vi "监控电脑运行信息vi.vi"() -> ()   [LabVIEW 2025]
uses:
  <vilib>/nisyscfg/File System.ctl
  <vilib>/nisyscfg/Access Point.ctl
  <vilib>/nisyscfg/Wireless Network.ctl
  <vilib>/nisyscfg/Resource Expert Info.ctl
  <resource>/objmgr/nicontrollersysapi.rc
  <resource>/objmgr/nisysapi.rc
  <vilib>/nisyscfg/nisyscfg.lvlib
panel:
  out "输出簇 2":T4 {"网络适配器:无线:发现接入点"."wireless network"."security type" items=["无"=0, "开环"=2, "WEP"=4, "WPA Personal"=8, "WPA Enterprise"=16, "WPA2 Personal"=32, "WPA2 Enterprise"=64]; "网络适配器:无线:发现接入点"."wireless network"."connection type" items=["无", "基础结构", "ad hoc"]; "网络适配器:无线:发现接入点"."link speed" items=["无"=0, "自适应"=1, "10mbps/半双工"=2, "10mbps/全双工"=4, "100mbps/半双工"=8, "100mbps/全双工"=16, "Gigabit/半双工"=32, "Gigabit/全双工"=64, "WLAN 802.11a"=131072, "WLAN 802.11b"=262144, "WLAN 802.11g"=524288, "WLAN 802.11n"=1048576, "WLAN 802.11n (5GHz)"=2097152]}
  in  "簇 2":T4={"系统硬件输出"=refnum, "错误输出"={"status"=FALSE, "code"=0, "source"=""}, "Startup Settings:Enable Secure Shell Server"=FALSE, "Startup Settings:Disable RT Startup App"=FALSE, "Startup Settings:Enable UI Desktop Environment"=FALSE, "Startup Settings:Enable LabVIEW Project Access"=FALSE, "属于设备"=FALSE, "属于机箱"=FALSE, "服务类型"=[], "设备与机箱:连接至总线类型"=0, "设备与机箱:提供总线类型"=0, "设备与机箱:供应商名称"="", "设备与机箱:产品名称"="", "设备与机箱:型号名称号"=0, "设备与机箱:序列号"="", "设备与机箱:属于NI产品"=FALSE, "设备与机箱:属于仿真"=FALSE, "设备与机箱:连接至链接名称"="", "设备与机箱:提供链接名称"="", "设备与机箱:插槽连接数"=0, "设备与机箱:提供插槽数"=0, "设备与机箱:插槽号"=0, "设备与机箱:插槽左偏移"=0, "设备与机箱:当前温度"=0.0, "设备与机箱:硬件版本"="", "设备与机箱:包含驱动"=-1, "设备与机箱:已存在"=-2, "设备与机箱:总线特定:供应商ID"=0, "设备与机箱:总线特定:产品ID"=0, "设备与机箱:总线特定:PXI/PCI总线数"=0, "设备与机箱:总线特定:PXI/PCI设备数"=0, "设备与机箱:总线特定:PXI/PCI函数数"=0, "设备与机箱:总线特定:PXI/PCI实际链接宽度"=0, "设备与机箱:总线特定:PXI/PCI最大链接宽度"=0, "设备与机箱:总线特定:USB接口"=0, "设备与机箱:总线特定:TCP/IP主机名称"="", "设备与机箱:总线特定:TCP/IP MAC地址"="", "设备与机箱:总线特定:TCP/IP地址"="", "设备与机箱:总线特定:TCP/IP设备类"="", "设备与机箱:总线特定:GPIB主地址"=0, "设备与机箱:总线特定:GPIB次地址"=0, "设备与机箱:总线特定:串行COM端口绑定"="", "设备与机箱:总线特定:cRIO模块编程模式"=0, "设备与机箱:外部校准:支持外部校准"=FALSE, "设备与机箱:外部校准:支持校准写入"=FALSE, "设备与机箱:外部校准:校准注释"="", "设备与机箱:外部校准:外部校准日期"=timestamp(0 s since 1904-01-01), "设备与机箱:外部校准:外部校准调整日期"=timestamp(0 s since 1904-01-01), "设备与机箱:外部校准:外部校准温度"=0.0, "设备与机箱:外部校准:外部校准截止日期"=timestamp(0 s since 1904-01-01), "设备与机箱:外部校准:推荐校准间隔"=0, "设备与机箱:外部校准:外部校准有限"=FALSE, "设备与机箱:外部校准:校准Checksum"="", "设备与机箱:内部校准:支持内部校准"=FALSE, "设备与机箱:内部校准:内部校准有限"=FALSE, "设备与机箱:内部校准:范围内内部校准值"=FALSE, "设备与机箱:内部校准:内部校准详细信息计数"=0, "设备与机箱:内部校准:内部校准名称"=[], "设备与机箱:内部校准:内部校准日期"=[], "设备与机箱:内部校准:内部校准温度"=[], "设备与机箱:固件:固件版本"="", "设备与机箱:固件:支持固件更新"=FALSE, "设备与机箱:固件:固件更新模式"=0, "设备与机箱:固件:固件文件匹配模式"="", "设备与机箱:固件:可用固件版本"=[], "设备与机箱:功能激活:功能激活状态"=0, "设备和机箱:功能激活:已激活功能的数量"=0, "设备和机箱:功能激活:已激活功能的名称"=[], "设备和机箱:功能激活:已激活功能的ID"=[], "启动设置:用户指定型安全模式"=FALSE, "启动设置:启用控制台输出"=FALSE, "启动设置:IP重置"=FALSE, "网络适配器:适配器类型"=1, "网络适配器:MAC地址"="", "网络适配器:属于主适配器"=FALSE, "网络适配器:适配器模式"=1, "网络适配器:TCP/IP:IP地址请求模式"=1, "网络适配器:TCP/IP:IP地址"="", "网络适配器:TCP/IP:子网掩码"="", "网络适配器:TCP/IP:网关"="", "网络适配器:TCP/IP:DNS服务器"="", "网络适配器:TCP/IP:当前链接速度"=1, "网络适配器:TCP/IP:包检测"=1, "网络适配器:TCP/IP:轮询间隔"=0, "网络适配器:无线:发现接入点"=[], "网络适配器:无线:SSID"="", "网络适配器:无线:连接类型"=0, "网络适配器:无线:安全类型"=0, "网络适配器:无线:链接质量"=0, "网络适配器:无线:通道编号"=0, "网络适配器:无线:BSSID"="", "网络适配器:无线:国家代码"=0, "网络适配器:无线:认证类型"=0, "系统资源:主磁盘空间"=0.0, "系统资源:剩余主磁盘空间"=0.0, "系统资源:CPU:CPU核心数量"=0, "系统资源:CPU:CPU逻辑处理器数量"=0, "系统资源:CPU:模型"="", "系统资源:CPU:步进修订"=0, "系统资源:CPU:总负载"=[], "系统资源:CPU:中断负载"=[], "系统资源:CPU:速度"=[], "系统资源:风扇:数量"=0, "系统资源:风扇:名称"=[], "系统资源:风扇:读数"=[], "系统资源:内存:物理内存总数"=0.0, "系统资源:内存:剩余物理内存"=0.0, "系统资源:内存:最大可用内存块"=0.0, "系统资源:内存:虚拟内存总数"=0.0, "系统资源:内存:剩余虚拟内存"=0.0, "系统资源:功率传感器:数量"=0, "系统资源:功率传感器:名称"=[], "系统资源:功率传感器:读数"=[], "系统资源:功率传感器:高临界值"=[], "系统资源:温度传感器:数量"=0, "系统资源:温度传感器:名称"=[], "系统资源:温度传感器:读数"=[], "系统资源:温度传感器:低临界值"=[], "系统资源:温度传感器:高临界值"=[], "系统资源:User LED:数量"=0, "系统资源:User LED:名称"=[], "系统资源:User LED:状态"=[], "系统资源:用户开关:数量"=0, "系统资源:用户开关:名称"=[], "系统资源:用户开关:状态"=[], "系统资源:电压传感器:数量"=0, "系统资源:电压传感器:名称"=[], "系统资源:电压传感器:读数"=[], "系统资源:电压传感器:额定值"=[], "系统资源:电压传感器:低临界值"=[], "系统资源:电压传感器:高临界值"=[], "时间:系统开始时间"=timestamp(0 s since 1904-01-01), "时间:当前时间"=timestamp(0 s since 1904-01-01), "时间:时区"="", "专项软件信息:专项软件名称"="", "专项软件信息:资源名称"="", "专项软件信息:用户别名"="", "专项软件信息:全部专项软件"=[], "System Resources:Memory Module:Location"=[], "System Resources:Memory Module:Model Name"=[], "System Resources:Memory Module:Capacity"=[], "System Resources:Fans:PXI Chassis Fan Control:Fan Mode"=1, "System Resources:Fans:PXI Chassis Fan Control:Fan User RPM"=0, "System Resources:Fans:PXI Chassis Fan Control:Fan User Duty Cycle"=0, "System Resources:Fans:PXI Chassis Fan Control:Fan User RPM Low Bound"=0, "System Resources:Fans:PXI Chassis Fan Control:Fan User RPM High Bound"=0, "System Resources:Fans:PXI Chassis Fan Control:Cooling Profile"=1, "System Resources:Fans:PXI Chassis Fan Control:Cooling Profile Source"=-1, "System Resources:Fans:PXI Chassis Fan Control:Enable User Override of Cooling Profile"=FALSE, "System Resources:Power Supplies:Count"=0, "System Resources:Power Supplies:Redundant"=0, "System Resources:Power Supplies:Bay Names"=[], "System Resources:Power Supplies:State"=[], "System Resources:Power Supplies:Max Power"=[], "System Resources:Power Supplies:Power Reading"=[], "System Resources:Power Supplies:Intake Temperature"=[], "System Resources:Power Supplies:Power Line Frequency"=[], "System Resources:Power Supplies:Inhibit Mode"=1, "Devices & Chassis:Bus Specific:PXI Chassis Number"=0, "Devices & Chassis:Bus Specific:PXI CLK10 Source"=-1, "Devices & Chassis:Bus Specific:External Clock Output Source"=-1, "Devices & Chassis:Bus Specific:Internal Oscillator"=-1, "Devices & Chassis:Bus Specific:High Density Trig Ports:Count"=0, "Devices & Chassis:Bus Specific:High Density Trig Ports:Names"=[], "Devices & Chassis:Bus Specific:High Density Trig Ports:States"=[], "Devices & Chassis:Bus Specific:High Density Trig Ports:Remote Aliases"=[], "Devices & Chassis:Bus Specific:Chassis LED Blink Pattern"=1, "Devices & Chassis:Calibration:PXI Chassis External Calibration Action"=0, "Devices & Chassis:Calibration:PXI Chassis Oscillator DAC Value"=0} {"Devices & Chassis:Calibration:PXI Chassis External Calibration Action" items=["Cancel", "OCXO Start", "Commit"]; "Devices & Chassis:Bus Specific:Chassis LED Blink Pattern" items=["Chassis Controlled"=1, "Blink"=2, "Blink | Blink | Blink"=4, "Blink | Blink | Steady"=8, "Blink | Steady | Blink"=16, "Blink | Steady | Steady"=32, "Steady | Blink | Blink"=64, "Steady | Blink | Steady"=128, "Steady | Steady | Blink"=256]; "Devices & Chassis:Bus Specific:High Density Trig Ports:States" items=["Disconnected", "Connected", "Connected (Off-Host)", "Loopback (Invalid)"]; "Devices & Chassis:Bus Specific:Internal Oscillator" items=["Unsupported"=-1, "VCXO"=0, "OCXO"=1]; "Devices & Chassis:Bus Specific:External Clock Output Source" items=["Unknown"=-1, "PXI_CLK10"=0, "Internal Oscillator"=1]; "Devices & Chassis:Bus Specific:PXI CLK10 Source" items=["Unknown"=-1, "Internal"=0, "10 MHz REF IN"=1, "Timing Module"=2, "TRIG / 10 MHz Port 0"=3]; "System Resources:Power Supplies:Inhibit Mode" items=["Default (Power Button/OS)"=1, "Manual (Remote Inhibit)"=2]; "System Resources:Power Supplies:State" items=["Off"=0, "On"=1, "Faulted"=2, "Fault: 12V Output Voltage Exceeded Upper Critical Limit"=16, "Fault: 12V Output Voltage Exceeded Lower Critical Limit"=17, "Fault: 5V Aux Output Voltage Exceeded Upper Critical Limit"=18, "Fault: 5V Aux Output Voltage Exceeded Lower Critical Limit"=19, "Fault: 12V Output Current Exceeded Critical Limit"=20, "Fault: 5V Aux Output Current Exceeded Critical Limit"=21, "Fault: AC Input Voltage Exceeded Upper Critical Limit"=22, "Fault: AC Input Voltage Exceeded Lower Critical Limit"=23, "Fault: Intake Temperature Exceeded Lower Critical Limit"=24, "Fault: Intake Temperature Exceeded Upper Critical Limit"=25, "Fault: Internal Temperature Exceeded Lower Critical Limit"=26, "Fault: Internal Temperature Exceeded Upper Critical Limit"=27, "Fault: Critical Fan Failure"=28, "Alert: 12V Output Voltage Exceeded Upper Alert Limit"=48, "Alert: 12V Output Voltage Exceeded Lower Alert Limit"=49, "Alert: 5V Aux Output Voltage Exceeded Upper Alert Limit"=50, "Alert: 5V Aux Output Voltage Exceeded Lower Alert Limit"=51, "Alert: 12V Output Current Exceeded Alert Limit"=52, "Alert: 5V Aux Output Current Exceeded Alert Limit"=53, "Alert: Current Sharing"=54, "Alert: AC Input Voltage Exceeded Upper Alert Limit"=55, "Alert: AC Input Voltage Exceeded Lower Alert Limit"=56, "Alert: Intake Temperature Exceeded Lower Alert Limit"=57, "Alert: Intake Temperature Exceeded Upper Alert Limit"=58, "Alert: Internal Temperature Exceeded Lower Alert Limit"=59, "Alert: Internal Temperature Exceeded Upper Alert Limit"=60, "Alert: Fan Failure"=61]; "System Resources:Power Supplies:Redundant" items=["Not Redundant", "Redundant"]; "System Resources:Fans:PXI Chassis Fan Control:Cooling Profile Source" items=["Unknown"=-1, "User Specified"=1, "Module Request"=2, "User Override of Module Request"=3]; "System Resources:Fans:PXI Chassis Fan Control:Cooling Profile" items=["38W"=1, "58W"=2, "82W"=4]; "System Resources:Fans:PXI Chassis Fan Control:Fan Mode" items=["Auto"=1, "Safe Manual"=2, "High"=4]; "系统资源:用户开关:状态" items=["Disabled", "已启用"]; "系统资源:User LED:状态" items=["Off"=0, "绿灯常亮"=1, "黄灯常亮"=2, "红灯常亮"=16, "绿灯闪烁"=4, "黄灯闪烁"=8, "红灯闪烁"=32]; "网络适配器:无线:认证类型" items=["None"=0, "EAP-TLS"=1, "EAP-TTLS"=2, "EAP-FAST"=4, "LEAP"=8, "PEAP"=16]; "网络适配器:无线:安全类型" items=["None"=0, "不支持"=1, "打开"=2, "WEP"=4, "WPA PSK"=8, "WPA EAP"=16, "WPA2 PSK"=32, "WPA2 EAP"=64]; "网络适配器:无线:连接类型" items=["None", "基础结构", "Ad Hoc"]; "网络适配器:无线:发现接入点"."wireless network"."security type" items=["无"=0, "开环"=2, "WEP"=4, "WPA Personal"=8, "WPA Enterprise"=16, "WPA2 Personal"=32, "WPA2 Enterprise"=64]; "网络适配器:无线:发现接入点"."wireless network"."connection type" items=["无", "基础结构", "ad hoc"]; "网络适配器:无线:发现接入点"."link speed" items=["无"=0, "自适应"=1, "10mbps/半双工"=2, "10mbps/全双工"=4, "100mbps/半双工"=8, "100mbps/全双工"=16, "Gigabit/半双工"=32, "Gigabit/全双工"=64, "WLAN 802.11a"=131072, "WLAN 802.11b"=262144, "WLAN 802.11g"=524288, "WLAN 802.11n"=1048576, "WLAN 802.11n (5GHz)"=2097152]; "网络适配器:TCP/IP:包检测" items=["Line Interrupt"=1, "轮询"=2, "消息信号中断"=4]; "网络适配器:TCP/IP:当前链接速度" items=["Autonegotiate"=1, "10 Mbps/半双工"=2, "10 Mbps/全双工"=4, "100 Mbps/半双工"=8, "100 Mbps/全双工"=16, "Gigabit/半双工"=32, "Gigabit/全双工"=64, "WLAN 802.11a"=131072, "WLAN 802.11b"=262144, "WLAN 802.11g"=524288, "WLAN 802.11n"=1048576, "WLAN 802.11n (5GHz)"=2097152]; "网络适配器:TCP/IP:IP地址请求模式" items=["Static"=1, "DHCP/Link Local"=2, "仅Link-Local"=4, "仅DHCP"=8]; "网络适配器:适配器模式" items=["Disabled"=1, "TCP/IP Ethernet"=2, "确定性"=4, "EtherCAT"=8, "TCP/IP WLAN连接"=32, "TCP/IP WLAN创建"=64]; "网络适配器:适配器类型" items=["Ethernet"=1, "WLAN"=2]; "设备与机箱:功能激活:功能激活状态" items=["None", "未激活", "已激活"]; "设备与机箱:固件:固件更新模式" items=["无", "手动", "驱动器管理"]; "设备与机箱:总线特定:cRIO模块编程模式" items=["None"=0, "Real-Time CPU"=1, "Real-Time扫描引擎"=2, "LabVIEW FPGA"=4]; "设备与机箱:已存在" items=["Initializing"=-2, "未知"=-1, "不存在"=0, "存在"=1]; "设备与机箱:包含驱动" items=["Unknown"=-1, "未安装"=0, "已安装"=1]; "设备与机箱:提供总线类型" items=["BuiltIn/System", "PXI/PCI", "USB", "GPIB", "VXI", "串行", "TCP/IP", "cRIO", "SCXI", "cDAQ", "SwitchBlock", "SCC", "FireWire", "附件", "CAN", "SwitchBlock设备", "SLSC"]; "设备与机箱:连接至总线类型" items=["BuiltIn/System", "PXI/PCI", "USB", "GPIB", "VXI", "串行", "TCP/IP", "cRIO", "SCXI", "cDAQ", "SwitchBlock", "SCC", "FireWire", "附件", "CAN", "SwitchBlock设备", "SLSC"]; "服务类型" items=["NI Network Resource", "NI Real-Time", "NI系统配置", "NI网络接口", "本地系统", "本地网络适配器", "本地计时器", "本地时间参考", "LXI仪器", "本地FPGA", "设备网络适配器"]}
  out "输出簇":T6 {"Real-Time:文件系统" items=["Default"=0, "FAT"=1, "Reliance"=2, "UBIFS"=16384, "Ext4"=32768]}
  in  "簇":T6={"系统资源:CPU:CPU逻辑处理器数量"=0, "设备类"="", "固件版本"="", "主机名称"="", "产品ID"=0, "产品名称"="", "序列号"="", "用户注释"="", "高级:自动重启超时"=0, "高级:存储位置"="", "高级:已安装的API版本"="", "镜像元数据:标题"="", "镜像元数据:说明"="", "镜像元数据:ID"="", "镜像元数据:版本"="", "操作系统:架构"="", "操作系统:版本"="", "操作系统:说明"="", "主NIC:DNS服务器"="", "主NIC:网关"="", "主NIC:IP地址"="", "主NIC:IP地址请求模式"=1, "主NIC:MAC地址"="", "主NIC:子网掩码"="", "Real-Time:文件系统"=0, "Real-Time:锁定"=FALSE, "Real-Time:支持锁定"=FALSE, "Real-Time:位于本地子网"=FALSE, "Real-Time:保护重启"=FALSE, "Real-Time:IP失败时中止"=FALSE, "Real-Time:支持重启"=FALSE, "Real-Time:系统状态"="", "系统资源:物理内存总数"=0.0, "系统资源:剩余物理内存"=0.0, "系统资源:最大可用内存块"=0.0, "系统资源:虚拟内存总数"=0.0, "系统资源:剩余虚拟内存"=0.0, "系统资源:主磁盘空间"=0.0, "系统资源:剩余主磁盘空间"=0.0} {"Real-Time:文件系统" items=["Default"=0, "FAT"=1, "Reliance"=2, "UBIFS"=16384, "Ext4"=32768]; "主NIC:IP地址请求模式" items=["Static"=1, "DHCP/Link-Local"=2, "仅Link-Local"=4, "仅DHCP"=8]}
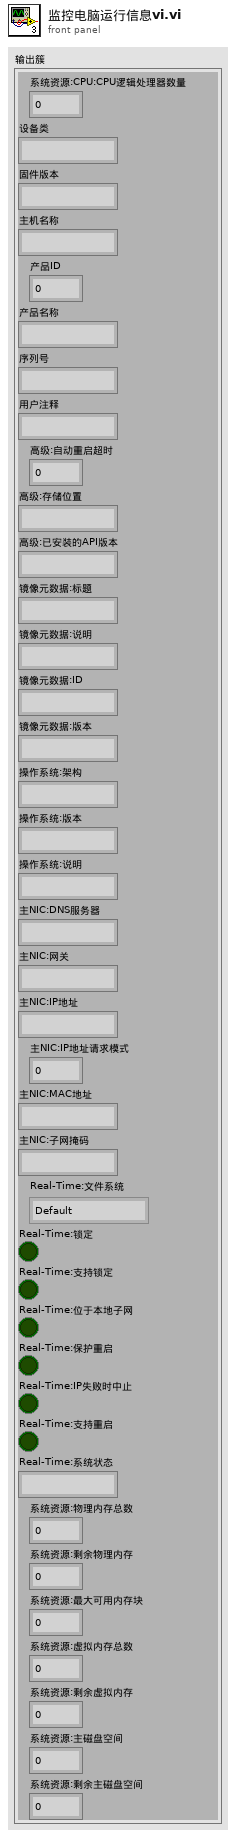
[diagram p1: front panel]
types:
  T1 = typedef "nisyscfg.lvlib/Access Point.ctl" = cluster{"wireless network":T2, "BSSID":string, "link quality":u32, "channel number":u32, "link speed":u32}
  T2 = typedef "nisyscfg.lvlib/Wireless Network.ctl" = cluster{"SSID":string, "connection type":u32, "security type":u32}
  T3 = typedef "nisyscfg.lvlib/Resource Expert Info.ctl" = cluster{"expert programmatic name":string, "expert-assigned resource name":string, "user-assigned alias":string}
  T4 = cluster{"系统硬件输出":refnum<k20>, "错误输出":errorcluster, "Startup Settings:Enable Secure Shell Server":bool, "Startup Settings:Disable RT Startup App":bool, "Startup Settings:Enable UI Desktop Environment":bool, "Startup Settings:Enable LabVIEW Project Access":bool, "属于设备":bool, "属于机箱":bool, "服务类型":u32[], "设备与机箱:连接至总线类型":u32, "设备与机箱:提供总线类型":u32, "设备与机箱:供应商名称":string, "设备与机箱:产品名称":string, "设备与机箱:型号名称号":u32, "设备与机箱:序列号":string, "设备与机箱:属于NI产品":bool, "设备与机箱:属于仿真":bool, "设备与机箱:连接至链接名称":string, "设备与机箱:提供链接名称":string, "设备与机箱:插槽连接数":i32, "设备与机箱:提供插槽数":i32, "设备与机箱:插槽号":i32, "设备与机箱:插槽左偏移":u32, "设备与机箱:当前温度":dbl, "设备与机箱:硬件版本":string, "设备与机箱:包含驱动":i32, "设备与机箱:已存在":i32, "设备与机箱:总线特定:供应商ID":u32, "设备与机箱:总线特定:产品ID":u32, "设备与机箱:总线特定:PXI/PCI总线数":u32, "设备与机箱:总线特定:PXI/PCI设备数":u32, "设备与机箱:总线特定:PXI/PCI函数数":u32, "设备与机箱:总线特定:PXI/PCI实际链接宽度":i32, "设备与机箱:总线特定:PXI/PCI最大链接宽度":i32, "设备与机箱:总线特定:USB接口":u32, "设备与机箱:总线特定:TCP/IP主机名称":string, "设备与机箱:总线特定:TCP/IP MAC地址":string, "设备与机箱:总线特定:TCP/IP地址":string, "设备与机箱:总线特定:TCP/IP设备类":string, "设备与机箱:总线特定:GPIB主地址":i32, "设备与机箱:总线特定:GPIB次地址":i32, "设备与机箱:总线特定:串行COM端口绑定":string, "设备与机箱:总线特定:cRIO模块编程模式":u32, "设备与机箱:外部校准:支持外部校准":bool, "设备与机箱:外部校准:支持校准写入":bool, "设备与机箱:外部校准:校准注释":string, "设备与机箱:外部校准:外部校准日期":timestamp, "设备与机箱:外部校准:外部校准调整日期":timestamp, "设备与机箱:外部校准:外部校准温度":dbl, "设备与机箱:外部校准:外部校准截止日期":timestamp, "设备与机箱:外部校准:推荐校准间隔":i32, "设备与机箱:外部校准:外部校准有限":bool, "设备与机箱:外部校准:校准Checksum":string, "设备与机箱:内部校准:支持内部校准":bool, "设备与机箱:内部校准:内部校准有限":bool, "设备与机箱:内部校准:范围内内部校准值":bool, "设备与机箱:内部校准:内部校准详细信息计数":i32, "设备与机箱:内部校准:内部校准名称":string[], "设备与机箱:内部校准:内部校准日期":timestamp[], "设备与机箱:内部校准:内部校准温度":dbl[], "设备与机箱:固件:固件版本":string, "设备与机箱:固件:支持固件更新":bool, "设备与机箱:固件:固件更新模式":u32, "设备与机箱:固件:固件文件匹配模式":string, "设备与机箱:固件:可用固件版本":string[], "设备与机箱:功能激活:功能激活状态":u32, "设备和机箱:功能激活:已激活功能的数量":u32, "设备和机箱:功能激活:已激活功能的名称":string[], "设备和机箱:功能激活:已激活功能的ID":u32[], "启动设置:用户指定型安全模式":bool, "启动设置:启用控制台输出":bool, "启动设置:IP重置":bool, "网络适配器:适配器类型":u32, "网络适配器:MAC地址":string, "网络适配器:属于主适配器":bool, "网络适配器:适配器模式":u32, "网络适配器:TCP/IP:IP地址请求模式":u32, "网络适配器:TCP/IP:IP地址":string, "网络适配器:TCP/IP:子网掩码":string, "网络适配器:TCP/IP:网关":string, "网络适配器:TCP/IP:DNS服务器":string, "网络适配器:TCP/IP:当前链接速度":u32, "网络适配器:TCP/IP:包检测":u32, "网络适配器:TCP/IP:轮询间隔":u32, "网络适配器:无线:发现接入点":T1[], "网络适配器:无线:SSID":string, "网络适配器:无线:连接类型":u32, "网络适配器:无线:安全类型":u32, "网络适配器:无线:链接质量":u32, "网络适配器:无线:通道编号":u32, "网络适配器:无线:BSSID":string, "网络适配器:无线:国家代码":i32, "网络适配器:无线:认证类型":u32, "系统资源:主磁盘空间":dbl, "系统资源:剩余主磁盘空间":dbl, "系统资源:CPU:CPU核心数量":i32, "系统资源:CPU:CPU逻辑处理器数量":i32, "系统资源:CPU:模型":string, "系统资源:CPU:步进修订":i32, "系统资源:CPU:总负载":u32[], "系统资源:CPU:中断负载":u32[], "系统资源:CPU:速度":u32[], "系统资源:风扇:数量":i32, "系统资源:风扇:名称":string[], "系统资源:风扇:读数":u32[], "系统资源:内存:物理内存总数":dbl, "系统资源:内存:剩余物理内存":dbl, "系统资源:内存:最大可用内存块":dbl, "系统资源:内存:虚拟内存总数":dbl, "系统资源:内存:剩余虚拟内存":dbl, "系统资源:功率传感器:数量":i32, "系统资源:功率传感器:名称":string[], "系统资源:功率传感器:读数":dbl[], "系统资源:功率传感器:高临界值":dbl[], "系统资源:温度传感器:数量":i32, "系统资源:温度传感器:名称":string[], "系统资源:温度传感器:读数":dbl[], "系统资源:温度传感器:低临界值":dbl[], "系统资源:温度传感器:高临界值":dbl[], "系统资源:User LED:数量":i32, "系统资源:User LED:名称":string[], "系统资源:User LED:状态":u32[], "系统资源:用户开关:数量":i32, "系统资源:用户开关:名称":string[], "系统资源:用户开关:状态":u32[], "系统资源:电压传感器:数量":i32, "系统资源:电压传感器:名称":string[], "系统资源:电压传感器:读数":dbl[], "系统资源:电压传感器:额定值":dbl[], "系统资源:电压传感器:低临界值":dbl[], "系统资源:电压传感器:高临界值":dbl[], "时间:系统开始时间":timestamp, "时间:当前时间":timestamp, "时间:时区":string, "专项软件信息:专项软件名称":string, "专项软件信息:资源名称":string, "专项软件信息:用户别名":string, "专项软件信息:全部专项软件":T3[], "System Resources:Memory Module:Location":string[], "System Resources:Memory Module:Model Name":string[], "System Resources:Memory Module:Capacity":dbl[], "System Resources:Fans:PXI Chassis Fan Control:Fan Mode":u32, "System Resources:Fans:PXI Chassis Fan Control:Fan User RPM":u32, "System Resources:Fans:PXI Chassis Fan Control:Fan User Duty Cycle":u32, "System Resources:Fans:PXI Chassis Fan Control:Fan User RPM Low Bound":u32, "System Resources:Fans:PXI Chassis Fan Control:Fan User RPM High Bound":u32, "System Resources:Fans:PXI Chassis Fan Control:Cooling Profile":u32, "System Resources:Fans:PXI Chassis Fan Control:Cooling Profile Source":i32, "System Resources:Fans:PXI Chassis Fan Control:Enable User Override of Cooling Profile":bool, "System Resources:Power Supplies:Count":i32, "System Resources:Power Supplies:Redundant":u32, "System Resources:Power Supplies:Bay Names":string[], "System Resources:Power Supplies:State":u32[], "System Resources:Power Supplies:Max Power":u32[], "System Resources:Power Supplies:Power Reading":dbl[], "System Resources:Power Supplies:Intake Temperature":dbl[], "System Resources:Power Supplies:Power Line Frequency":u32[], "System Resources:Power Supplies:Inhibit Mode":u32, "Devices & Chassis:Bus Specific:PXI Chassis Number":u32, "Devices & Chassis:Bus Specific:PXI CLK10 Source":i32, "Devices & Chassis:Bus Specific:External Clock Output Source":i32, "Devices & Chassis:Bus Specific:Internal Oscillator":i32, "Devices & Chassis:Bus Specific:High Density Trig Ports:Count":i32, "Devices & Chassis:Bus Specific:High Density Trig Ports:Names":string[], "Devices & Chassis:Bus Specific:High Density Trig Ports:States":u32[], "Devices & Chassis:Bus Specific:High Density Trig Ports:Remote Aliases":string[], "Devices & Chassis:Bus Specific:Chassis LED Blink Pattern":u32, "Devices & Chassis:Calibration:PXI Chassis External Calibration Action":u32, "Devices & Chassis:Calibration:PXI Chassis Oscillator DAC Value":u32}
  T5 = typedef "nisyscfg.lvlib/File System.ctl" = i32
  T6 = cluster{"系统资源:CPU:CPU逻辑处理器数量":i32, "设备类":string, "固件版本":string, "主机名称":string, "产品ID":i32, "产品名称":string, "序列号":string, "用户注释":string, "高级:自动重启超时":u32, "高级:存储位置":string, "高级:已安装的API版本":string, "镜像元数据:标题":string, "镜像元数据:说明":string, "镜像元数据:ID":string, "镜像元数据:版本":string, "操作系统:架构":string, "操作系统:版本":string, "操作系统:说明":string, "主NIC:DNS服务器":string, "主NIC:网关":string, "主NIC:IP地址":string, "主NIC:IP地址请求模式":i32, "主NIC:MAC地址":string, "主NIC:子网掩码":string, "Real-Time:文件系统":T5, "Real-Time:锁定":bool, "Real-Time:支持锁定":bool, "Real-Time:位于本地子网":bool, "Real-Time:保护重启":bool, "Real-Time:IP失败时中止":bool, "Real-Time:支持重启":bool, "Real-Time:系统状态":string, "系统资源:物理内存总数":dbl, "系统资源:剩余物理内存":dbl, "系统资源:最大可用内存块":dbl, "系统资源:虚拟内存总数":dbl, "系统资源:剩余虚拟内存":dbl, "系统资源:主磁盘空间":dbl, "系统资源:剩余主磁盘空间":dbl}
  T7 = typedef "File System.ctl" = i32
  T8 = typedef "Access Point.ctl" = cluster{"wireless network":T2, "BSSID":string, "link quality":u32, "channel number":u32, "link speed":u32}
  T9 = typedef "Resource Expert Info.ctl" = cluster{"expert programmatic name":string, "expert-assigned resource name":string, "user-assigned alias":string}
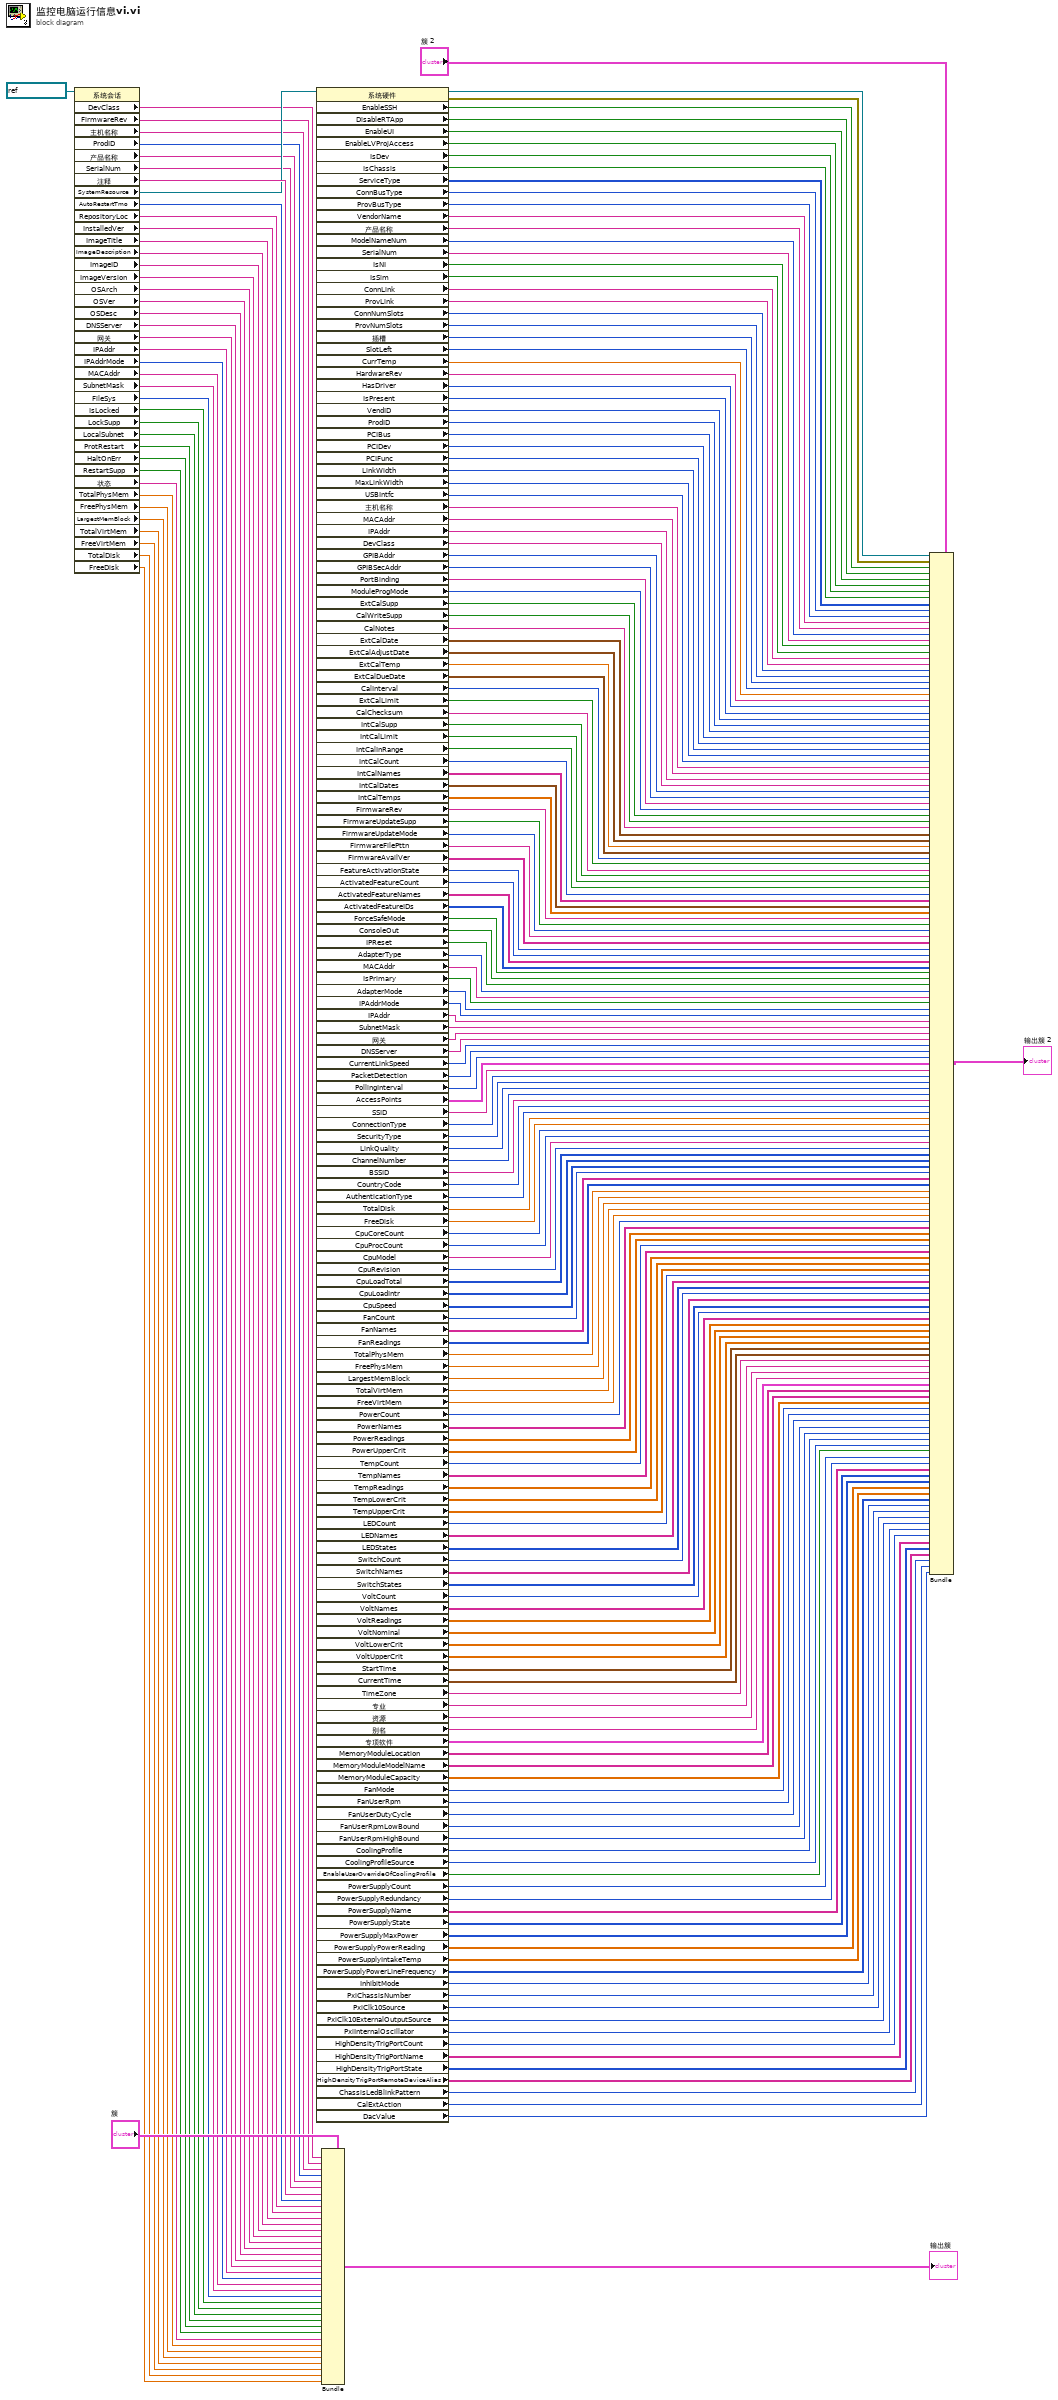
[diagram p0: block diagram]
diagram:
  n1 = property class="系统会话"(reference=refnum<k21> "localhost" ("Target (localhost)")) -> ("DevClass"=w172:string, "FirmwareRev"=w173:string, "主机名称"=w174:string, "ProdID"=w175:i32, "产品名称"=w176:string, "SerialNum"=w177:string, "注释"=w179:string, "SystemResource"=w178:refnum<k20>, "AutoRestartTmo"=w180:u32, "RepositoryLoc"=w181:string, "InstalledVer"=w182:string, "ImageTitle"=w183:string, "ImageDescription"=w184:string, "ImageID"=w185:string, "ImageVersion"=w186:string, "OSArch"=w187:string, "OSVer"=w188:string, "OSDesc"=w189:string, "DNSServer"=w190:string, "网关"=w191:string, "IPAddr"=w192:string, "IPAddrMode"=w193:i32, "MACAddr"=w194:string, "SubnetMask"=w195:string, "FileSys"=w196:T7, "IsLocked"=w197:bool, "LockSupp"=w198:bool, "LocalSubnet"=w199:bool, "ProtRestart"=w200:bool, "HaltOnErr"=w201:bool, "RestartSupp"=w203:bool, "状态"=w202:string, "TotalPhysMem"=w210:dbl, "FreePhysMem"=w209:dbl, "LargestMemBlock"=w208:dbl, "TotalVirtMem"=w207:dbl, "FreeVirtMem"=w206:dbl, "TotalDisk"=w205:dbl, "FreeDisk"=w204:dbl)  [unwired: 1 in, 2 out]
  n2 = property class="系统硬件"(reference=w178) -> (reference out=w170:refnum<k20>, error out=w169:errorcluster, "EnableSSH"=w168:bool, "DisableRTApp"=w167:bool, "EnableUI"=w166:bool, "EnableLVProjAccess"=w165:bool, "IsDev"=w164:bool, "IsChassis"=w163:bool, "ServiceType"=w162:u32[], "ConnBusType"=w161:u32, "ProvBusType"=w160:u32, "VendorName"=w159:string, "产品名称"=w158:string, "ModelNameNum"=w157:u32, "SerialNum"=w156:string, "IsNI"=w155:bool, "IsSim"=w154:bool, "ConnLink"=w153:string, "ProvLink"=w152:string, "ConnNumSlots"=w151:i32, "ProvNumSlots"=w150:i32, "插槽"=w149:i32, "SlotLeft"=w148:u32, "CurrTemp"=w147:dbl, "HardwareRev"=w146:string, "HasDriver"=w145:i32, "IsPresent"=w144:i32, "VendID"=w143:u32, "ProdID"=w142:u32, "PCIBus"=w141:u32, "PCIDev"=w140:u32, "PCIFunc"=w139:u32, "LinkWidth"=w138:i32, "MaxLinkWidth"=w137:i32, "USBIntfc"=w136:u32, "主机名称"=w135:string, "MACAddr"=w134:string, "IPAddr"=w133:string, "DevClass"=w132:string, "GPIBAddr"=w131:i32, "GPIBSecAddr"=w130:i32, "PortBinding"=w129:string, "ModuleProgMode"=w128:u32, "ExtCalSupp"=w127:bool, "CalWriteSupp"=w126:bool, "CalNotes"=w125:string, "ExtCalDate"=w124:timestamp, "ExtCalAdjustDate"=w123:timestamp, "ExtCalTemp"=w122:dbl, "ExtCalDueDate"=w121:timestamp, "CalInterval"=w120:i32, "ExtCalLimit"=w119:bool, "CalChecksum"=w118:string, "IntCalSupp"=w117:bool, "IntCalLimit"=w116:bool, "IntCalInRange"=w115:bool, "IntCalCount"=w114:i32, "IntCalNames"=w113:string[], "IntCalDates"=w112:timestamp[], "IntCalTemps"=w111:dbl[], "FirmwareRev"=w110:string, "FirmwareUpdateSupp"=w109:bool, "FirmwareUpdateMode"=w108:u32, "FirmwareFilePttn"=w107:string, "FirmwareAvailVer"=w106:string[], "FeatureActivationState"=w105:u32, "ActivatedFeatureCount"=w104:u32, "ActivatedFeatureNames"=w103:string[], "ActivatedFeatureIDs"=w102:u32[], "ForceSafeMode"=w101:bool, "ConsoleOut"=w100:bool, "IPReset"=w99:bool, "AdapterType"=w98:u32, "MACAddr"=w97:string, "IsPrimary"=w96:bool, "AdapterMode"=w94:u32, "IPAddrMode"=w95:u32, "IPAddr"=w93:string, "SubnetMask"=w92:string, "网关"=w91:string, "DNSServer"=w90:string, "CurrentLinkSpeed"=w89:u32, "PacketDetection"=w88:u32, "PollingInterval"=w87:u32, "AccessPoints"=w86:T8[], "SSID"=w85:string, "ConnectionType"=w84:u32, "SecurityType"=w83:u32, "LinkQuality"=w82:u32, "ChannelNumber"=w81:u32, "BSSID"=w80:string, "CountryCode"=w78:i32, "AuthenticationType"=w79:u32, "TotalDisk"=w77:dbl, "FreeDisk"=w76:dbl, "CpuCoreCount"=w75:i32, "CpuProcCount"=w74:i32, "CpuModel"=w73:string, "CpuRevision"=w72:i32, "CpuLoadTotal"=w71:u32[], "CpuLoadIntr"=w70:u32[], "CpuSpeed"=w69:u32[], "FanCount"=w68:i32, "FanNames"=w67:string[], "FanReadings"=w66:u32[], "TotalPhysMem"=w65:dbl, "FreePhysMem"=w64:dbl, "LargestMemBlock"=w63:dbl, "TotalVirtMem"=w62:dbl, "FreeVirtMem"=w61:dbl, "PowerCount"=w60:i32, "PowerNames"=w59:string[], "PowerReadings"=w58:dbl[], "PowerUpperCrit"=w57:dbl[], "TempCount"=w56:i32, "TempNames"=w55:string[], "TempReadings"=w54:dbl[], "TempLowerCrit"=w53:dbl[], "TempUpperCrit"=w52:dbl[], "LEDCount"=w51:i32, "LEDNames"=w50:string[], "LEDStates"=w49:u32[], "SwitchCount"=w48:i32, "SwitchNames"=w47:string[], "SwitchStates"=w46:u32[], "VoltCount"=w45:i32, "VoltNames"=w44:string[], "VoltReadings"=w43:dbl[], "VoltNominal"=w42:dbl[], "VoltLowerCrit"=w41:dbl[], "VoltUpperCrit"=w40:dbl[], "StartTime"=w39:timestamp, "CurrentTime"=w38:timestamp, "TimeZone"=w37:string, "专业"=w36:string, "资源"=w35:string, "别名"=w34:string, "专项软件"=w33:T9[], "MemoryModuleLocation"=w32:string[], "MemoryModuleModelName"=w31:string[], "MemoryModuleCapacity"=w30:dbl[], "FanMode"=w29:u32, "FanUserRpm"=w28:u32, "FanUserDutyCycle"=w27:u32, "FanUserRpmLowBound"=w26:u32, "FanUserRpmHighBound"=w25:u32, "CoolingProfile"=w24:u32, "CoolingProfileSource"=w23:i32, "EnableUserOverrideOfCoolingProfile"=w22:bool, "PowerSupplyCount"=w21:i32, "PowerSupplyRedundancy"=w20:u32, "PowerSupplyName"=w19:string[], "PowerSupplyState"=w18:u32[], "PowerSupplyMaxPower"=w17:u32[], "PowerSupplyPowerReading"=w16:dbl[], "PowerSupplyIntakeTemp"=w15:dbl[], "PowerSupplyPowerLineFrequency"=w14:u32[], "InhibitMode"=w13:u32, "PxiChassisNumber"=w12:u32, "PxiClk10Source"=w11:i32, "PxiClk10ExternalOutputSource"=w10:i32, "PxiInternalOscillator"=w9:i32, "HighDensityTrigPortCount"=w8:i32, "HighDensityTrigPortName"=w7:string[], "HighDensityTrigPortState"=w6:u32[], "HighDensityTrigPortRemoteDeviceAlias"=w5:string[], "ChassisLedBlinkPattern"=w4:u32, "CalExtAction"=w3:u32, "DacValue"=w2:u32)  [unwired: 1 in]
  n3 = Bundle(cluster="簇", "设备类"=w172, "固件版本"=w173, "主机名称"=w174, "产品ID"=w175, "产品名称"=w176, "序列号"=w177, "用户注释"=w179, "高级:自动重启超时"=w180, "高级:存储位置"=w181, "高级:已安装的API版本"=w182, "镜像元数据:标题"=w183, "镜像元数据:说明"=w184, "镜像元数据:ID"=w185, "镜像元数据:版本"=w186, "操作系统:架构"=w187, "操作系统:版本"=w188, "操作系统:说明"=w189, "主NIC:DNS服务器"=w190, "主NIC:网关"=w191, "主NIC:IP地址"=w192, "主NIC:IP地址请求模式"=w193, "主NIC:MAC地址"=w194, "主NIC:子网掩码"=w195, "Real-Time:文件系统"=w196, "Real-Time:锁定"=w197, "Real-Time:支持锁定"=w198, "Real-Time:位于本地子网"=w199, "Real-Time:保护重启"=w200, "Real-Time:IP失败时中止"=w201, "Real-Time:支持重启"=w203, "Real-Time:系统状态"=w202, "系统资源:物理内存总数"=w210, "系统资源:剩余物理内存"=w209, "系统资源:最大可用内存块"=w208, "系统资源:虚拟内存总数"=w207, "系统资源:剩余虚拟内存"=w206, "系统资源:主磁盘空间"=w205, "系统资源:剩余主磁盘空间"=w204) -> (→"输出簇":T6)  [unwired: 1 in]
  n4 = Bundle(cluster="簇 2", "系统硬件输出"=w170, "错误输出"=w169, "Startup Settings:Enable Secure Shell Server"=w168, "Startup Settings:Disable RT Startup App"=w167, "Startup Settings:Enable UI Desktop Environment"=w166, "Startup Settings:Enable LabVIEW Project Access"=w165, "属于设备"=w164, "属于机箱"=w163, "服务类型"=w162, "设备与机箱:连接至总线类型"=w161, "设备与机箱:提供总线类型"=w160, "设备与机箱:供应商名称"=w159, "设备与机箱:产品名称"=w158, "设备与机箱:型号名称号"=w157, "设备与机箱:序列号"=w156, "设备与机箱:属于NI产品"=w155, "设备与机箱:属于仿真"=w154, "设备与机箱:连接至链接名称"=w153, "设备与机箱:提供链接名称"=w152, "设备与机箱:插槽连接数"=w151, "设备与机箱:提供插槽数"=w150, "设备与机箱:插槽号"=w149, "设备与机箱:插槽左偏移"=w148, "设备与机箱:当前温度"=w147, "设备与机箱:硬件版本"=w146, "设备与机箱:包含驱动"=w145, "设备与机箱:已存在"=w144, "设备与机箱:总线特定:供应商ID"=w143, "设备与机箱:总线特定:产品ID"=w142, "设备与机箱:总线特定:PXI/PCI总线数"=w141, "设备与机箱:总线特定:PXI/PCI设备数"=w140, "设备与机箱:总线特定:PXI/PCI函数数"=w139, "设备与机箱:总线特定:PXI/PCI实际链接宽度"=w138, "设备与机箱:总线特定:PXI/PCI最大链接宽度"=w137, "设备与机箱:总线特定:USB接口"=w136, "设备与机箱:总线特定:TCP/IP主机名称"=w135, "设备与机箱:总线特定:TCP/IP MAC地址"=w134, "设备与机箱:总线特定:TCP/IP地址"=w133, "设备与机箱:总线特定:TCP/IP设备类"=w132, "设备与机箱:总线特定:GPIB主地址"=w131, "设备与机箱:总线特定:GPIB次地址"=w130, "设备与机箱:总线特定:串行COM端口绑定"=w129, "设备与机箱:总线特定:cRIO模块编程模式"=w128, "设备与机箱:外部校准:支持外部校准"=w127, "设备与机箱:外部校准:支持校准写入"=w126, "设备与机箱:外部校准:校准注释"=w125, "设备与机箱:外部校准:外部校准日期"=w124, "设备与机箱:外部校准:外部校准调整日期"=w123, "设备与机箱:外部校准:外部校准温度"=w122, "设备与机箱:外部校准:外部校准截止日期"=w121, "设备与机箱:外部校准:推荐校准间隔"=w120, "设备与机箱:外部校准:外部校准有限"=w119, "设备与机箱:外部校准:校准Checksum"=w118, "设备与机箱:内部校准:支持内部校准"=w117, "设备与机箱:内部校准:内部校准有限"=w116, "设备与机箱:内部校准:范围内内部校准值"=w115, "设备与机箱:内部校准:内部校准详细信息计数"=w114, "设备与机箱:内部校准:内部校准名称"=w113, "设备与机箱:内部校准:内部校准日期"=w112, "设备与机箱:内部校准:内部校准温度"=w111, "设备与机箱:固件:固件版本"=w110, "设备与机箱:固件:支持固件更新"=w109, "设备与机箱:固件:固件更新模式"=w108, "设备与机箱:固件:固件文件匹配模式"=w107, "设备与机箱:固件:可用固件版本"=w106, "设备与机箱:功能激活:功能激活状态"=w105, "设备和机箱:功能激活:已激活功能的数量"=w104, "设备和机箱:功能激活:已激活功能的名称"=w103, "设备和机箱:功能激活:已激活功能的ID"=w102, "启动设置:用户指定型安全模式"=w101, "启动设置:启用控制台输出"=w100, "启动设置:IP重置"=w99, "网络适配器:适配器类型"=w98, "网络适配器:MAC地址"=w97, "网络适配器:属于主适配器"=w96, "网络适配器:适配器模式"=w94, "网络适配器:TCP/IP:IP地址请求模式"=w95, "网络适配器:TCP/IP:IP地址"=w93, "网络适配器:TCP/IP:子网掩码"=w92, "网络适配器:TCP/IP:网关"=w91, "网络适配器:TCP/IP:DNS服务器"=w90, "网络适配器:TCP/IP:当前链接速度"=w89, "网络适配器:TCP/IP:包检测"=w88, "网络适配器:TCP/IP:轮询间隔"=w87, "网络适配器:无线:发现接入点"=w86, "网络适配器:无线:SSID"=w85, "网络适配器:无线:连接类型"=w84, "网络适配器:无线:安全类型"=w83, "网络适配器:无线:链接质量"=w82, "网络适配器:无线:通道编号"=w81, "网络适配器:无线:BSSID"=w80, "网络适配器:无线:国家代码"=w78, "网络适配器:无线:认证类型"=w79, "系统资源:主磁盘空间"=w77, "系统资源:剩余主磁盘空间"=w76, "系统资源:CPU:CPU核心数量"=w75, "系统资源:CPU:CPU逻辑处理器数量"=w74, "系统资源:CPU:模型"=w73, "系统资源:CPU:步进修订"=w72, "系统资源:CPU:总负载"=w71, "系统资源:CPU:中断负载"=w70, "系统资源:CPU:速度"=w69, "系统资源:风扇:数量"=w68, "系统资源:风扇:名称"=w67, "系统资源:风扇:读数"=w66, "系统资源:内存:物理内存总数"=w65, "系统资源:内存:剩余物理内存"=w64, "系统资源:内存:最大可用内存块"=w63, "系统资源:内存:虚拟内存总数"=w62, "系统资源:内存:剩余虚拟内存"=w61, "系统资源:功率传感器:数量"=w60, "系统资源:功率传感器:名称"=w59, "系统资源:功率传感器:读数"=w58, "系统资源:功率传感器:高临界值"=w57, "系统资源:温度传感器:数量"=w56, "系统资源:温度传感器:名称"=w55, "系统资源:温度传感器:读数"=w54, "系统资源:温度传感器:低临界值"=w53, "系统资源:温度传感器:高临界值"=w52, "系统资源:User LED:数量"=w51, "系统资源:User LED:名称"=w50, "系统资源:User LED:状态"=w49, "系统资源:用户开关:数量"=w48, "系统资源:用户开关:名称"=w47, "系统资源:用户开关:状态"=w46, "系统资源:电压传感器:数量"=w45, "系统资源:电压传感器:名称"=w44, "系统资源:电压传感器:读数"=w43, "系统资源:电压传感器:额定值"=w42, "系统资源:电压传感器:低临界值"=w41, "系统资源:电压传感器:高临界值"=w40, "时间:系统开始时间"=w39, "时间:当前时间"=w38, "时间:时区"=w37, "专项软件信息:专项软件名称"=w36, "专项软件信息:资源名称"=w35, "专项软件信息:用户别名"=w34, "专项软件信息:全部专项软件"=w33, "System Resources:Memory Module:Location"=w32, "System Resources:Memory Module:Model Name"=w31, "System Resources:Memory Module:Capacity"=w30, "System Resources:Fans:PXI Chassis Fan Control:Fan Mode"=w29, "System Resources:Fans:PXI Chassis Fan Control:Fan User RPM"=w28, "System Resources:Fans:PXI Chassis Fan Control:Fan User Duty Cycle"=w27, "System Resources:Fans:PXI Chassis Fan Control:Fan User RPM Low Bound"=w26, "System Resources:Fans:PXI Chassis Fan Control:Fan User RPM High Bound"=w25, "System Resources:Fans:PXI Chassis Fan Control:Cooling Profile"=w24, "System Resources:Fans:PXI Chassis Fan Control:Cooling Profile Source"=w23, "System Resources:Fans:PXI Chassis Fan Control:Enable User Override of Cooling Profile"=w22, "System Resources:Power Supplies:Count"=w21, "System Resources:Power Supplies:Redundant"=w20, "System Resources:Power Supplies:Bay Names"=w19, "System Resources:Power Supplies:State"=w18, "System Resources:Power Supplies:Max Power"=w17, "System Resources:Power Supplies:Power Reading"=w16, "System Resources:Power Supplies:Intake Temperature"=w15, "System Resources:Power Supplies:Power Line Frequency"=w14, "System Resources:Power Supplies:Inhibit Mode"=w13, "Devices & Chassis:Bus Specific:PXI Chassis Number"=w12, "Devices & Chassis:Bus Specific:PXI CLK10 Source"=w11, "Devices & Chassis:Bus Specific:External Clock Output Source"=w10, "Devices & Chassis:Bus Specific:Internal Oscillator"=w9, "Devices & Chassis:Bus Specific:High Density Trig Ports:Count"=w8, "Devices & Chassis:Bus Specific:High Density Trig Ports:Names"=w7, "Devices & Chassis:Bus Specific:High Density Trig Ports:States"=w6, "Devices & Chassis:Bus Specific:High Density Trig Ports:Remote Aliases"=w5, "Devices & Chassis:Bus Specific:Chassis LED Blink Pattern"=w4, "Devices & Chassis:Calibration:PXI Chassis External Calibration Action"=w3, "Devices & Chassis:Calibration:PXI Chassis Oscillator DAC Value"=w2) -> (→"输出簇 2":T4)
